vi "Process data measurement.vi"(8 "Error in":errorcluster, 9 "I-V Graph history":cluster{"Voltage (V)":dbl, "Current (A)":dbl}[](array[cluster]), 11 "Byte array":u8[](array[numeric])) -> (0 "Error out":errorcluster, 3 "I-V Graph":cluster{"Voltage (V)":dbl, "Current (A)":dbl}[](array[cluster]))   [LabVIEW 2020]
uses:
  Typedefs/Measurement data.ctl
  COBS/COBS.lvlib
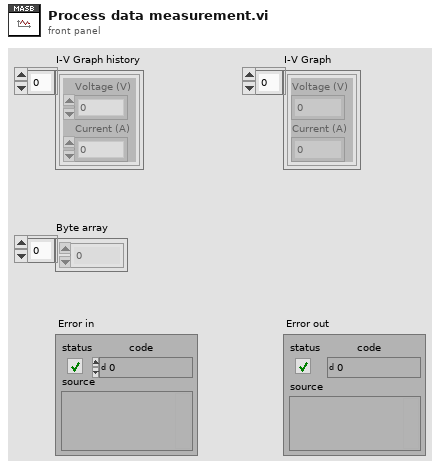
[diagram p1: front panel]
types:
  T1 = typedef "Measurement data.ctl" = cluster{"Point":u32, "Time (ms)":u32, "Voltage (V)":dbl, "Current (A)":dbl}
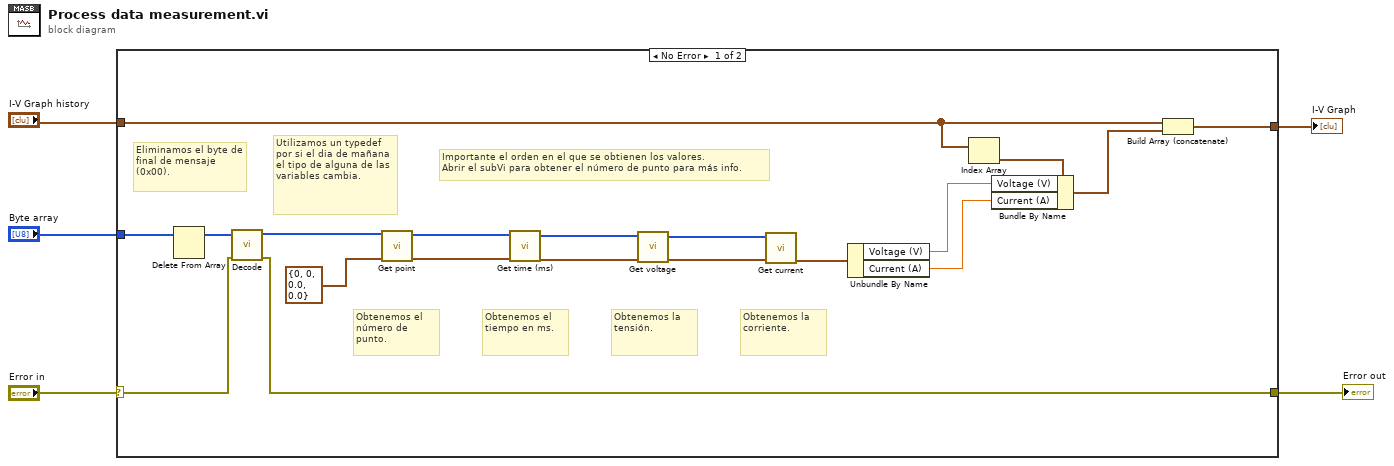
[diagram p0: block diagram]
diagram:
  n1 = case shown="No Error" "Error in" {
    selector: "Error in" -> [w7 w26]
    tunnel: [w6 w26] -> w5
    tunnel: [w24 w25] -> w3
    tunnel: "I-V Graph history" -> [w23 w25]
    tunnel: "Byte array" -> [w20 _]
    frame No Error {
      # "Utilizamos un typedef por si el dia de mañana el tipo de alguna de las variables cambia."
      # "Importante el orden en el que se obtienen los valores.\nAbrir el subVi para obtener el número de punto para más info."
      # "Obtenemos la corriente."
      # "Obtenemos la tensión."
      # "Obtenemos el tiempo en ms."
      # "Obtenemos el número de punto."
      # "Eliminamos el byte de final de mensaje (0x00)."
      n2 = Delete From Array(array=w20) -> (array with subset deleted=w9:u8[])  [unwired: 2 in, 1 out]
      n3 = call "Decode.vi"("Error in"=w7, "Encoded message"=w9) -> ("Error out"=w6:errorcluster, "Decoded message"=w8:u8[])  [unwired: 8 in]
      n4 = call "Get point.vi"("Measurement data in"=T1 {"Point"=0, "Time (ms)"=0, "Voltage (V)"=0.0, "Current (A)"=0.0} ("Measurement data"), "Byte array"=w8) -> ("Measurement data out"=w17:T1, "Byte array"=w18:u8[])  [unwired: 8 in]
      n5 = call "Get time (ms).vi"("Measurement data in"=w17, "Byte array"=w18) -> ("Measurement data out"=w15:T1, "Byte array"=w16:u8[])  [unwired: 8 in]
      n6 = call "Get voltage.vi"("Measurement data in"=w15, "Byte array"=w16) -> ("Measurement data out"=w13:T1, "Byte array"=w14:u8[])  [unwired: 8 in]
      n7 = call "Get current.vi"("Measurement data in"=w13, "Byte array"=w14) -> ("Measurement data out"=w12:T1)  [unwired: 8 in, 1 out]
      n8 = Unbundle By Name(w12) -> ("Voltage (V)"=w11:dbl, "Current (A)"=w10:dbl)
      n9 = Index Array(array=w23) -> (element=w22:cluster{"Voltage (V)":dbl, "Current (A)":dbl})  [unwired: 1 in]
      n10 = Bundle By Name(cluster=w22, "Voltage (V)"=w11, "Current (A)"=w10) -> (w21:cluster{"Voltage (V)":dbl, "Current (A)":dbl})
      n11 = Build Array (concatenate)(w23, w21) -> (w24:cluster{"Voltage (V)":dbl, "Current (A)":dbl}[])
    }
    frame Error {
    }
  }
  "Error out" <- w5
  "I-V Graph" <- w3
